vi "FAMM-Save-TAG_property_record.vi"(8 "error in (no error)":errorcluster, 9 "TAG-property":T1 {"TAGprop"."TagFunc" format="%08x"; "TAGprop"."RangeL" format="%.2f"; "TAGprop"."RangeH" format="%.2f"}, 10 "Source":string, 11 "FAMM in":refnum<class "FAMM.lvclass">) -> (0 "error out":errorcluster, 3 "FAMM out":refnum<class "FAMM.lvclass">)   [LabVIEW 2020, in "Sgraph_lib_V1.lvlib" / "FAMM.lvclass"]
doc: "Andre Koelewijn, 18 aug 2021\n\nSave one TAG propertie from the DB editor utility."
uses:
  FAMM.lvclass
  DBAL/controls/DBAL_TAGpropEdit.ctl
  Common/controls/typedef_com_TagProp.ctl
  Gserver/controls/Typedef_QueryType.ctl
  FAMM.lvclass/FAMM.ctl
  <vilib>/Utility/error.llb/Error Cluster From Error Code.vi
  <vilib>/ErrorRing/Error Ring.xnode
  DBAL/DBAL.lvclass
  Gserver/Gserver.lvclass
  Builds/Sgraph_lib_V1.lvlib
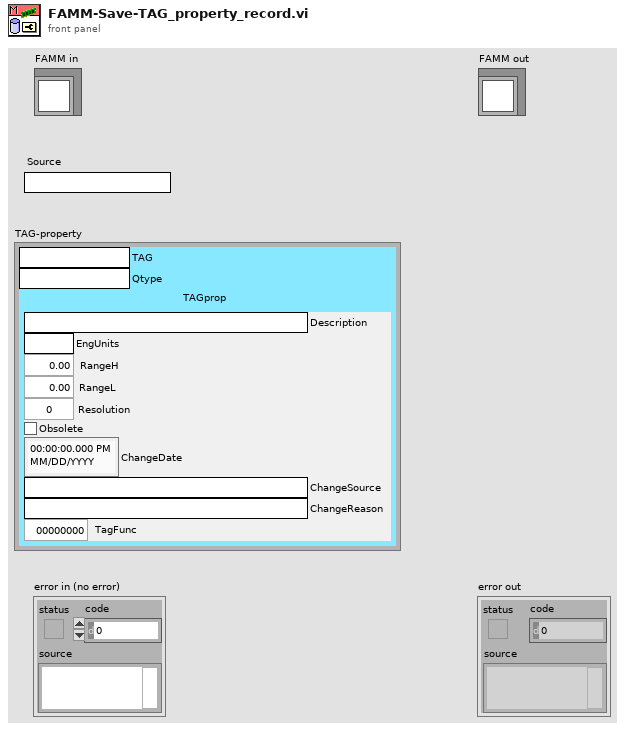
[diagram p1: front panel]
types:
  T1 = typedef "Sgraph_lib_V1.lvlib/DBAL.lvclass/DBAL_TAGpropEdit.ctl" = cluster{"TAG":string, "Qtype":string, "TAGprop":T2}
  T2 = typedef "Sgraph_lib_V1.lvlib/typedef_com_TagProp.ctl" = cluster{"Description":string, "EngUnits":string, "RangeH":dbl, "RangeL":dbl, "Resolution":i32, "Obsolete":bool, "ChangeDate":timestamp, "ChangeSource":string, "ChangeReason":string, "TagFunc":u32}
  T3 = typedef "Sgraph_lib_V1.lvlib/Gserver.lvclass/Typedef_QueryType.ctl" = enum16{"Subscribe", "DataRequest", "RequestAllTags", "RequestIniPath", "FAMMstarted", "SetClientOptions", "GviewerUpdate", "OpenNewGraph", "CloseClient", "CloseAllClients", "Close Gserver", "OpenMemoryMap", "MeMapDataRequest", "MeMapDataResponse", "OpenDBeditor", "CheckDBeditorRunning", "StoppedDBeditor", "SaveDB_TAGpropRecord", "ConfirmDB_TAGpropSave"}
  T4 = typedef "Sgraph_lib_V1.lvlib/FAMM.lvclass/FAMM-attributes.ctl" = cluster{"FAMM_PAQ_Layers":i32, "FAMM_PAQ_resolution":dbl, "PAQ_TAGs":string[], "WAQ_TAGs":string[], "EAQ_TAGs":string[], "All_TAGs":string[], "PAQtagProps":T2[], "WAQtagProps":T2[], "EAQtagProps":T2[], "DBAL_class":refnum<data-value>, "PAQ_memory":refnum<data-value>[], "PAQupdates":timestamp[], "FAMM_Size":cluster{"other":i32, "1day":i32, "1week":i32}, "DatabaseFileExtention":string, "DatabaseSaveRate":dbl, "Database_path":path, "DBAL-Queue":refnum<queue>, "OS_name":string}
  T5 = typedef "Sgraph_lib_V1.lvlib/DBAL.lvclass/DBAL_TAGprops.ctl" = T1[]
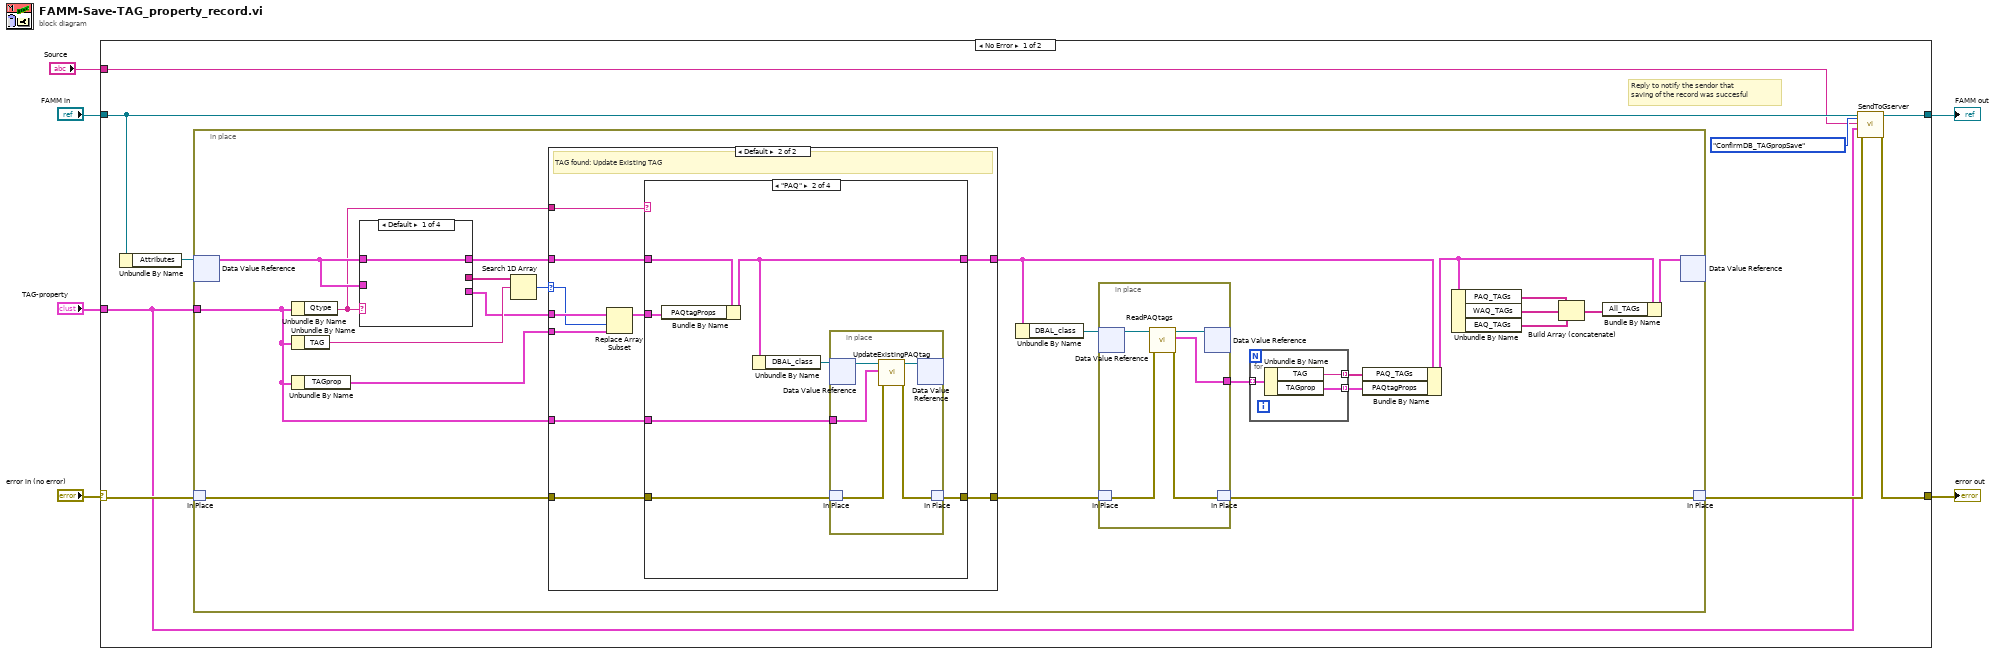
[diagram p0: block diagram]
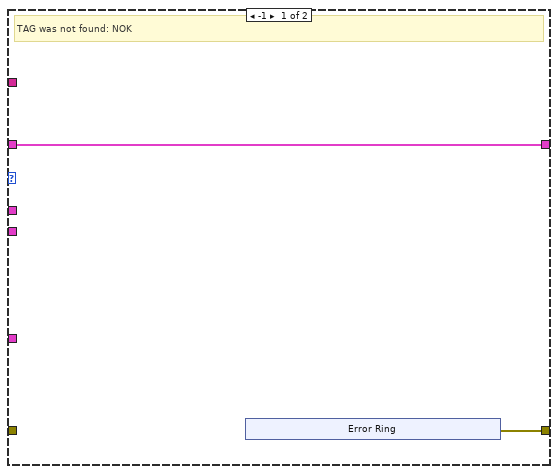
[diagram p2: hidden frame]
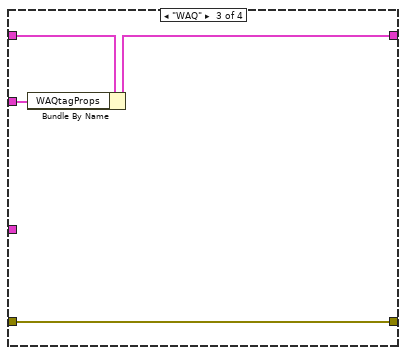
[diagram p4: hidden frame]
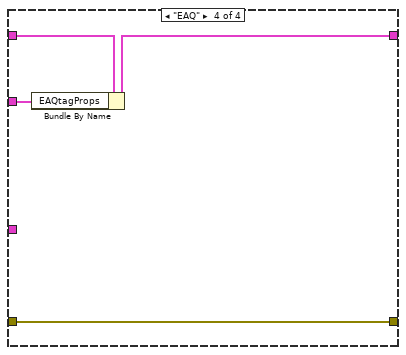
[diagram p5: hidden frame]
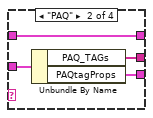
[diagram p6: hidden frame]
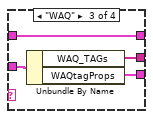
[diagram p7: hidden frame]
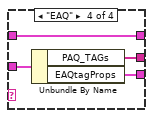
[diagram p8: hidden frame]
diagram:
  n1 = case shown="No Error" "error in (no error)" {
    selector: "error in (no error)" -> [w14 w100]
    tunnel: [w9 w100] -> w5
    tunnel: [w12 w99] -> w3
    tunnel: "FAMM in" -> [w11 w99]
    tunnel: "TAG-property" -> [w7 _]
    tunnel: "Source" -> [w8 _]
    frame No Error {
      # "Reply to notify the sendor that\nsaving of the record was succesful"
      n2 = Unbundle By Name(w11) -> ("Attributes"=w15:refnum<data-value>)
      n3 = in-place {
        in-place-border: w7 -> [w29]
        n4 = in-place-dvr #1(w15) -> (w33:T4)  [unwired: 1 out]
        n5 = in-place-match #2(w14) -> (w30:errorcluster)
        n6 = Unbundle By Name(w29) -> ("Qtype"=w32:string)
        n7 = Unbundle By Name(w29) -> ("TAG"=w37:string)
        n8 = Unbundle By Name(w29) -> ("TAGprop"=w34:T2)
        n9 = case shown="Default" w32 {
          tunnel: w33 -> [_ w90 w94 w98]
          tunnel: [_ w89 w93 w97] -> w36
          tunnel: [_ w88 w92 w96] -> w38
          tunnel: w33 -> [w86 w87 w91 w95]
          tunnel: [w86 w87 w91 w95] -> w31
          frame Default {
          }
          frame "PAQ" {
            n10 = Unbundle By Name(w90) -> ("PAQ_TAGs"=w88:string[], "PAQtagProps"=w89:T2[])
          }
          frame "WAQ" {
            n11 = Unbundle By Name(w94) -> ("WAQ_TAGs"=w92:string[], "WAQtagProps"=w93:T2[])
          }
          frame "EAQ" {
            n12 = Unbundle By Name(w98) -> ("PAQ_TAGs"=w96:string[], "EAQtagProps"=w97:T2[])
          }
        }
        n13 = Search 1D Array(1D array=w38, element=w37) -> (index of element=w35:i32)  [unwired: 1 in]
        n14 = case shown="Default" w35 {
          selector: w35 -> [_ w62]
          tunnel: w36 -> [_ w63]
          tunnel: w34 -> [_ w61]
          tunnel: w32 -> [_ w60]
          tunnel: w31 -> [w47 w59]
          tunnel: [w47 w57] -> w19
          tunnel: w30 -> [_ w56]
          tunnel: [w48 w55] -> w17
          tunnel: w29 -> [_ w54]
          frame -1 {
            # "TAG was not found: NOK"
            n15 = xnode "Error Ring"() -> ("error out"=w48:errorcluster)
          }
          frame Default {
            # "TAG found: Update Existing TAG"
            n16 = Replace Array Subset(array=w63, new element=w61, index=w62) -> (w58:T2[])
            n17 = case shown="\"PAQ\"" w60 {
              tunnel: w59 -> [w65 w72 w81 w85]
              tunnel: [w65 w70 w80 w83] -> w57
              tunnel: w58 -> [_ w71 w79 w84]
              tunnel: w56 -> [w64 w68 w78 w82]
              tunnel: [w64 w67 w78 w82] -> w55
              tunnel: w54 -> [_ w66 _ _]
              frame Default {
              }
              frame "PAQ" {
                n18 = Bundle By Name(cluster=w72, "PAQtagProps"=w71) -> (w70:T4)
                n19 = Unbundle By Name(w70) -> ("DBAL_class"=w69:refnum<data-value>)
                n20 = in-place {
                  in-place-border: w66 -> [w73]
                  n21 = in-place-dvr #3(w69) -> (w77:refnum<class "DBAL.lvclass">)  [unwired: 1 out]
                  n22 = in-place-match #4(w68) -> (w76:errorcluster)
                  n23 = call-dynamic "UpdateExistingPAQtag.vi"("error in (no error)"=w76, "TAGpropertyEdit"=w73, "DBAL in"=w77) -> ("error out"=w75:errorcluster, "DBAL out"=w74:refnum<class "DBAL.lvclass">)  [unwired: 7 in]
                  n24 = in-place-dvr #3(w74) -> ()  [unwired: 2 out]
                  n25 = in-place-match #4(w75) -> (w67:errorcluster)
                }
              }
              frame "WAQ" {
                n26 = Bundle By Name(cluster=w81, "WAQtagProps"=w79) -> (w80:T4)
              }
              frame "EAQ" {
                n27 = Bundle By Name(cluster=w85, "EAQtagProps"=w84) -> (w83:T4)
              }
            }
          }
        }
        n28 = Unbundle By Name(w19) -> ("DBAL_class"=w28:refnum<data-value>)
        n29 = in-place {
          in-place-border: [w42] -> w20
          n30 = in-place-dvr #5(w28) -> (w46:refnum<class "DBAL.lvclass">)  [unwired: 1 out]
          n31 = in-place-match #6(w17) -> (w45:errorcluster)
          n32 = call-dynamic "ReadPAQtags.vi"("error in (no error)"=w45, "DBAL in"=w46) -> ("error out"=w44:errorcluster, "PAQ_TAGs"=w42:T5, "DBAL out"=w43:refnum<class "DBAL.lvclass">)  [unwired: 7 in]
          n33 = in-place-dvr #5(w43) -> ()  [unwired: 2 out]
          n34 = in-place-match #6(w44) -> (w16:errorcluster)
        }
        n35 = for {
          tunnel: w20 -> [w41] mode=indexing
          tunnel: [w40] -> w21 mode=indexing
          tunnel: [w39] -> w22 mode=indexing
          n36 = Unbundle By Name(w41) -> ("TAG"=w40:string, "TAGprop"=w39:T2)
        }
        n37 = Bundle By Name(cluster=w19, "PAQ_TAGs"=w21, "PAQtagProps"=w22) -> (w27:T4)
        n38 = Unbundle By Name(w27) -> ("PAQ_TAGs"=w23:string[], "WAQ_TAGs"=w24:string[], "EAQ_TAGs"=w25:string[])
        n39 = Build Array (concatenate)(w23, w24, w25) -> (w26:string[])
        n40 = Bundle By Name(cluster=w27, "All_TAGs"=w26) -> (w18:T4)
        n41 = in-place-dvr #1(w18) -> ()  [unwired: 2 out]
        n42 = in-place-match #2(w16) -> (w10:errorcluster)
      }
      n43 = call "SendToGserver.vi"("Query_type"=Typedef_QueryType."ConfirmDB_TAGpropSave", "error in (no error)"=w10, "data"=w7, "Address"=w8, "FAMM in"=w11) -> ("error out"=w9:errorcluster, "FAMM out"=w12:refnum<class "FAMM.lvclass">)  [unwired: 5 in]
    }
    frame Error {
    }
  }
  "error out" <- w5
  "FAMM out" <- w3
